vi "Day 2-1.vi"() -> ()   [LabVIEW 2019, in "Day 2.lvlib"]
uses:
  <vilib>/Utility/error.llb/Error Cluster From Error Code.vi
  <vilib>/ErrorRing/Error Ring.xnode
  Day 2.lvlib
panel:
  out "error IO":errorcluster
  out "Result":u32
  out "Horizontal":u32
  out "Depth":i32
  out "Array 2":i32[](array[numeric])
  out "Array":string[](array[string])
  in  "String":string="forward 9\ndown 3\ndown 8\nforward 2\nup 3\nforward 5\nup 8\ndown 2\ndown 5\nup 7\ndown 9\nforward 4\nup 5\ndown 9\nforward 2\nforward 2\nforward 8\ndown 6\nforward 2\nup 9\nup 5\ndown 2\nforward 5\ndown 8\nforward 3\nup 4\nforward 5\nforward 7\ndown 8\ndown 6\nup 7\ndown 3\nforward 4\nup 8\ndown 5\ndown 3\ndown 6\ndown 8\nforward 1\nforward 9\nforward 4\nup 7\ndown 4\nforward 7\nforward 3\nforward 9\ndown 1\ndown 3\nup 9\ndown 3\nforward 9\nup 6\nup 9\ndown 8\nup 3\ndown 1\nup 8\ndown 8\ndown 2\ndown 4\ndown 4\nup 3\ndown 6\ndown 1\ndown 3\nforward 1\nup 5\nforward 5\nforward 8\ndown 2\nforward 6\nforward 2\nup 7\nforward 6\ndown 8\nforward 6\nforward 5\nup 9\nforward 5\nup 5\nforward 9\ndown 2\ndown 4\ndown 3\ndown 8\nforward 9\nforward 6\nforward 2\nup 7\ndown 7\nup 3\nforward 4\nforward 5\ndown 7\nforward 5\nup 9\nforward 6\nforward 6\nforward 1\ndown 6\nforward 9\nup 2\ndown 7\ndown 8\ndown 6\nup 5\ndown 8\ndown 8\nforward 7\ndown 6\nup 5\ndown 9\ndown 3\nforward 2\ndown 4\nforward 8\ndown 5\nup 5\nforward 7\nup 2\nup 2\ndown 4\nforward 4\ndown 5\nup 8\ndown 2\nforward 4\ndown 9\nforward 8\ndown 5\ndown 6\ndown 7\nup 7\nup 5\nup 7\nforward 7\nforward 8\ndown 2\nforward 3\ndown 2\ndown 7\ndown 4\ndown 2\nforward 3\nforward 5\ndown 3\ndown 7\nup 7\ndown 7\nup 5\nforward 1\ndown 8\ndown 2\nup 4\nup 5\ndown 8\nforward 9\ndown 3\ndown 9\nforward 8\nforward 1\nforward 1\ndown 2\nup 9\ndown 2\nup 8\ndown 6\nup 8\nforward 7\ndown 5\nforward 7\ndown 8\nforward 8\ndown 7\nup 9\nup 2\nup 6\ndown 5\ndown 9\nforward 2\nup 3\ndown 4\nup 5\nup 4\ndown 9\nforward 7\nforward 7\ndown 3\nforward 4\nforward 9\nup 8\nforward 3\ndown 1\nforward 2\ndown 7\ndown 3\ndown 7\ndown 7\nforward 8\nforward 4\nforward 7\nup 1\ndown 4\nup 9\ndown 2\ndown 1\nforward 6\ndown 3\nforward 7\nforward 8\nup 9\nup 2\nup 2\nforward 7\nup 2\nup 5\nforward 5\ndown 3\nforward 8\nforward 1\nup 4\ndown 6\ndown 5\nforward 4\nup 9\nforward 8\nup 4\ndown 8\ndown 3\ndown 3\ndown 7\nforward 2\nforward 4\ndown 9\ndown 7\ndown 2\nup 3\nup 3\nforward 8\nforward 7\nforward 8\ndown 5\nup 5\nforward 3\nforward 6\nup 7\nup 1\nforward 2\nforward 5\ndown 5\nforward 8\ndown 2\ndown 4\nforward 2\ndown 7\ndown 3\ndown 5\nforward 9\ndown 7\ndown 8\nup 1\nup 2\ndown 8\nforward 7\nforward 8\ndown 8\nforward 5\nup 7\nforward 3\nup 2\ndown 7\nforward 1\ndown 2\nup 7\nup 4\ndown 2\nforward 1\nup 5\nforward 2\nup 2\nforward 3\nforward 9\nforward 2\nforward 8\nforward 2\nup 7\ndown 8\ndown 7\nforward 2\nforward 7\ndown 1\nforward 2\nup 1\nup 6\ndown 3\ndown 6\nforward 7\ndown 4\nforward 5\nforward 6\nup 3\nforward 3\ndown 6\nforward 8\nup 8\nforward 4\ndown 3\nforward 3\ndown 4\ndown 7\nforward 9\nforward 2\nup 2\nforward 8\ndown 6\nforward 6\ndown 9\ndown 9\nforward 8\ndown 1\nforward 9\ndown 1\ndown 6\ndown 8\ndown 5\ndown 5\nforward 3\nforward 3\ndown 2\ndown 5\nforward 9\ndown 2\ndown 8\ndown 3\nforward 9\nup 2\ndown 4\ndown 9\nforward 9\nforward 1\nforward 5\nup 9\ndown 1\ndown 6\nforward 6\nforward 5\nforward 8\ndown 2\nforward 8\ndown 4\ndown 2\ndown 6\ndown 6\nup 3\nup 8\nforward 1\ndown 1\nup 8\ndown 3\ndown 4\nup 9\nup 1\ndown 7\ndown 7\nup 1\nup 2\nforward 5\nup 8\nforward 2\ndown 3\nforward 1\nup 5\nforward 6\nforward 2\ndown 6\nup 2\nforward 2\nforward 1\ndown 3\nforward 4\nup 8\nforward 5\ndown 4\nforward 2\ndown 8\ndown 7\nup 7\ndown 8\nforward 1\ndown 4\nup 9\ndown 6\nup 6\nup 6\ndown 2\nforward 1\nforward 8\ndown 6\nup 3\ndown 7\nforward 9\nup 1\nup 4\nforward 7\ndown 7\nforward 1\ndown 6\ndown 4\ndown 7\ndown 8\ndown 8\nforward 4\ndown 6\ndown 6\ndown 5\nforward 6\nup 9\nup 3\ndown 4\nforward 8\ndown 7\nforward 6\nup 3\nforward 1\nforward 1\ndown 8\nforward 7\nforward 4\nforward 6\nup 1\nforward 7\nup 8\nforward 2\nforward 6\nforward 8\ndown 9\ndown 8\nup 9\nup 4\nup 2\nforward 2\nforward 8\nup 2\nforward 3\nforward 2\nup 2\nup 5\nup 8\nforward 4\nforward 8\nforward 3\nup 5\ndown 1\nforward 2\ndown 7\ndown 8\nforward 3\nup 1\nforward 5\nforward 7\nforward 9\nup 7\nforward 4\ndown 4\nup 2\nforward 4\nforward 5\nforward 3\nup 9\nforward 6\nforward 8\ndown 9\ndown 1\nforward 1\ndown 5\ndown 2\nforward 9\ndown 2\nup 9\ndown 1\nforward 5\nforward 8\nup 2\nforward 6\ndown 4\ndown 9\nforward 4\nforward 1\ndown 3\ndown 3\nup 5\nforward 5\ndown 6\nforward 3\ndown 2\nforward 8\ndown 7\ndown 2\ndown 1\nforward 2\nup 5\nforward 9\nforward 3\nforward 5\ndown 4\nup 7\nforward 6\ndown 3\nforward 1\nforward 7\nforward 1\nup 4\ndown 2\ndown 7\nup 9\nforward 9\ndown 8\ndown 1\nup 2\ndown 3\nforward 7\ndown 8\ndown 5\ndown 5\nup 8\nforward 1\ndown 5\nforward 8\nup 7\ndown 1\nforward 9\ndown 4\nforward 8\nforward 5\nforward 7\nforward 8\nforward 3\nup 9\nforward 3\ndown 7\ndown 5\nup 8\nforward 3\nup 6\nforward 8\nup 3\ndown 5\nforward 5\nforward 6\nforward 4\nforward 3\nforward 8\nup 9\nforward 2\ndown 6\ndown 4\ndown 5\nforward 7\ndown 2\nup 5\nforward 2\nforward 5\ndown 9\nforward 8\ndown 8\nforward 6\ndown 9\ndown 7\nup 9\nforward 3\nforward 3\nup 5\ndown 2\nforward 5\ndown 6\ndown 6\ndown 2\ndown 3\ndown 4\nforward 7\nup 1\ndown 7\nforward 7\nup 1\nforward 3\nup 6\ndown 7\ndown 5\nforward 9\nforward 2\ndown 5\nforward 9\ndown 5\nforward 9\nforward 1\ndown 4\nforward 9\ndown 5\nforward 8\ndown 6\ndown 4\ndown 5\nforward 9\ndown 1\nforward 6\nforward 9\ndown 1\ndown 1\nup 2\nforward 5\nforward 3\ndown 4\nup 8\nforward 8\ndown 2\nforward 3\nforward 1\ndown 7\nforward 6\nforward 5\nup 7\nup 8\ndown 5\nup 3\ndown 8\nforward 6\nforward 5\nforward 6\nup 1\nup 8\nup 7\ndown 5\nforward 3\nforward 9\nup 9\nup 4\nup 7\nup 8\nforward 7\nforward 3\nforward 9\ndown 7\nforward 3\ndown 6\nforward 9\ndown 1\nforward 3\ndown 1\nforward 8\nforward 7\ndown 2\nforward 1\nforward 6\nforward 7\ndown 3\ndown 2\ndown 1\nforward 7\nforward 4\ndown 6\nup 4\nforward 4\nforward 9\nforward 3\ndown 1\nup 2\ndown 3\ndown 5\nforward 7\nforward 5\nup 1\ndown 2\ndown 3\ndown 8\nforward 1\ndown 4\nforward 5\ndown 5\nup 6\ndown 6\ndown 8\nforward 1\nforward 9\nup 5\nforward 2\ndown 9\ndown 5\ndown 1\ndown 4\ndown 9\ndown 8\nforward 2\nforward 4\nup 2\nforward 3\ndown 8\ndown 5\nup 5\nforward 8\nup 2\ndown 8\nup 3\nforward 7\ndown 7\nforward 8\ndown 7\ndown 3\nup 6\nforward 5\nup 4\nup 5\nforward 9\nforward 6\ndown 9\nforward 5\ndown 5\ndown 3\nforward 2\ndown 1\nup 9\nup 8\ndown 6\ndown 1\nforward 9\nforward 4\nforward 2\nup 1\nforward 5\nforward 9\nup 5\nforward 8\nforward 4\ndown 4\ndown 4\ndown 2\nforward 1\nforward 7\ndown 9\nforward 4\ndown 5\ndown 4\ndown 7\ndown 2\nforward 9\ndown 3\nforward 6\nforward 3\ndown 9\ndown 3\ndown 4\ndown 9\ndown 9\nup 6\ndown 5\nup 4\ndown 1\ndown 1\nforward 9\nforward 7\ndown 9\nforward 4\ndown 8\ndown 7\nforward 7\nforward 4\nup 2\nup 5\nforward 2\nforward 7\ndown 1\nforward 6\nforward 6\nforward 3\nforward 8\ndown 2\nup 2\nforward 7\nup 5\ndown 1\ndown 5\nforward 8\ndown 6\nforward 8\ndown 5\ndown 4\ndown 6\nforward 5\ndown 1\nforward 9\nforward 8\nup 5\ndown 6\nforward 5\nup 5\ndown 4\nforward 1\ndown 2\ndown 5\ndown 3\nforward 2\ndown 9\nforward 1\nforward 1\nforward 1\nforward 8\nforward 2\ndown 8\ndown 6\nup 1\nforward 6\ndown 3\ndown 4\nup 9\ndown 3\ndown 3\nup 7\ndown 4\nforward 4\nforward 9\ndown 3\ndown 8\nforward 5\ndown 3\ndown 6\ndown 7\nforward 1\nup 2\nforward 8\ndown 1\ndown 4\nup 9\nforward 9\nup 4\nup 2\nforward 3\nforward 4\ndown 2\ndown 2\ndown 6\nforward 6\nforward 8\ndown 6\nup 6\ndown 5\nforward 1\ndown 4\nup 9\nforward 1\nforward 3\ndown 1\ndown 4\nup 6\nforward 5\nforward 6\nup 9\nup 9\ndown 2\nup 6\nforward 1\nforward 2\nforward 3\nforward 3\nforward 6\nup 2\ndown 8\ndown 9\nforward 7\nup 1\nup 3\ndown 2\nforward 3\ndown 8\nforward 9\ndown 3\nforward 6\nup 2\nforward 7\ndown 2\nforward 5\ndown 4\ndown 2\nup 8\nforward 3\nforward 5\nforward 9\nforward 5\nforward 3\nup 9\ndown 7\nforward 4\nforward 2\nforward 7\ndown 5\nup 6\nup 6\nforward 8\ndown 2\nforward 1\nup 1\nup 9\nup 8\nup 3\nup 4\ndown 2\nup 7\ndown 4\nup 5\ndown 1\nup 9\ndown 5\ndown 9\ndown 4\nup 2\ndown 8\nup 2\nup 7\nup 9\nforward 4\nforward 2\nforward 1\nforward 6\nforward 8\nup 5\nforward 5\nforward 5\ndown 4\nup 6\nforward 3\ndown 9\ndown 7\nforward 4\ndown 3\nup 1\nforward 4\ndown 2\ndown 6\nup 3\nup 1\ndown 9\ndown 7\ndown 9\nforward 3\nforward 8\ndown 8\nup 7\nup 6\ndown 2\ndown 9\ndown 1\ndown 9\nforward 6\nup 4\ndown 3\nforward 5\nup 3\nup 9\nup 8\nforward 6\ndown 8\nforward 6\nforward 6\nforward 5\nup 4\ndown 4\nup 6\nup 4\nforward 2\ndown 5\nforward 9\nup 7\nup 6\ndown 4\nforward 7\nforward 6\nup 2\ndown 8\ndown 6\nforward 5\nup 2\nforward 5\nforward 1\nup 9\ndown 8\nforward 7\nup 4\nforward 8\ndown 4\nforward 3\nforward 3\ndown 9\nforward 4\nforward 9\nup 8\nforward 7\nforward 3\nforward 9\nforward 4\nup 3\nforward 2\nforward 7"
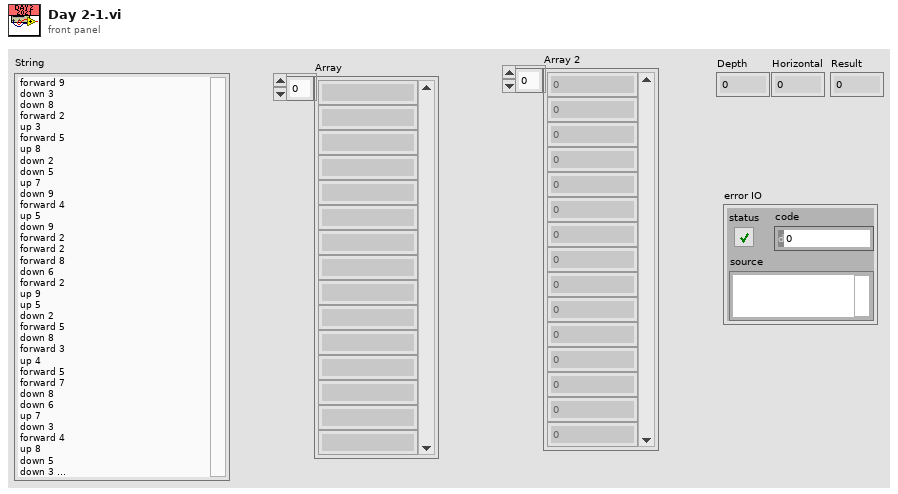
[diagram p1: front panel]
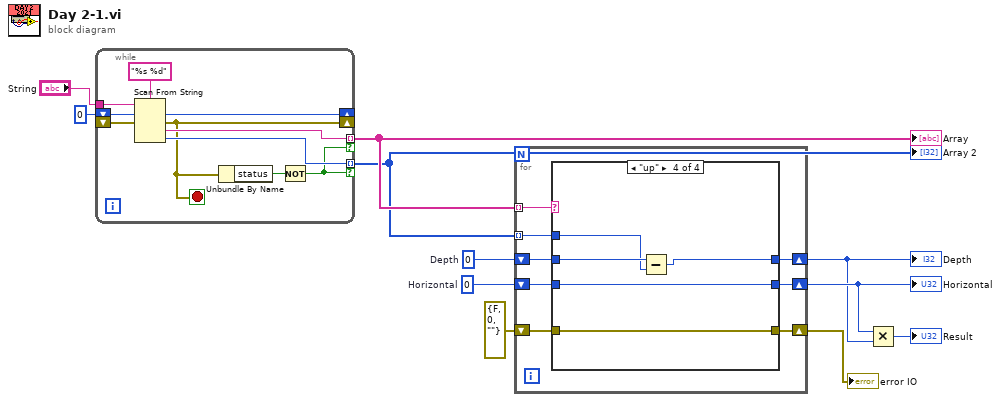
[diagram p0: block diagram]
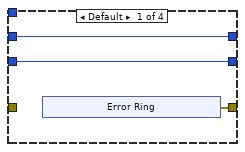
[diagram p2: hidden frame]
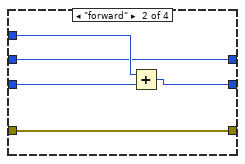
[diagram p3: hidden frame]
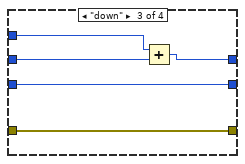
[diagram p4: hidden frame]
diagram:
  w7 = u32 0  # Horizontal
  w6 = 0  # Depth
  n1 = while {
    tunnel: [w19] -> w9 mode=indexing if=w12
    tunnel: [w18] -> w8 mode=indexing if=w12
    tunnel: "String" -> [w21]
    shift-right: [w15] -> _
    shift-left: u32 0 -> [w17]
    shift-right: [w14] -> _
    shift-left: _ -> [w16]
    stop <- w14 stop-if-true
    n2 = Scan From String(format string="%s %d", input string=w21, initial scan location=w17, error in=w16) -> (offset past scan=w15:u32, error out=w14:errorcluster, output 1=w19:string, output 2=w18:i32)  [unwired: 2 in, 1 out]
    n3 = Unbundle By Name(w14) -> ("status"=w13:bool)
    n4 = Not(x=w13) -> (.not. x?=w12:bool)
  }
  "Array" <- w9
  "Array 2" <- w8
  n5 = for {
    tunnel: w9 -> [w29] mode=indexing
    tunnel: w8 -> [w28] mode=indexing
    shift-right: [w26] -> w5
    shift-left: w7 -> [w22]
    shift-right: [w25] -> w4
    shift-left: w6 -> [w27]
    shift-right: [w24] -> w2
    shift-left: errorcluster {"status"=FALSE, "code"=0, "source"=""} ("error out") -> [w23]
    n6 = case shown="\"up\"" w29 {
      tunnel: w28 -> [_ w42 w47 w51]
      tunnel: w27 -> [w31 w39 w46 w52]
      tunnel: w22 -> [w30 w41 w44 w50]
      tunnel: [w30 w40 w44 w50] -> w26
      tunnel: [w31 w39 w45 w49] -> w25
      tunnel: [w32 w38 w43 w48] -> w24
      tunnel: w23 -> [_ w38 w43 w48]
      frame Default {
        n7 = xnode "Error Ring"() -> ("error out"=w32:errorcluster)
      }
      frame "forward" {
        n8 = Add(x=w42, y=w41) -> (x+y=w40:u32)
      }
      frame "down" {
        n9 = Add(x=w47, y=w46) -> (x+y=w45:i32)
      }
      frame "up" {
        n10 = Subtract(x=w52, y=w51) -> (x-y=w49:i32)
      }
    }
  }
  "Depth" <- w4
  "Horizontal" <- w5
  "error IO" <- w2
  n11 = Multiply(x=w5, y=w4) -> (x*y=→"Result":u32)
